vi "diffs.vi"(10 "Array":i32[](array[numeric])) -> (2 "Diffs":i32[](array[numeric]))   [LabVIEW 2014]
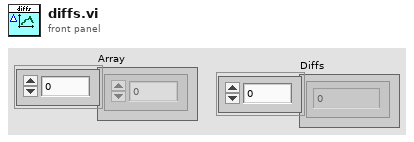
[diagram p1: front panel]
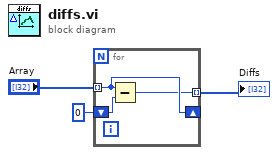
[diagram p0: block diagram]
diagram:
  n1 = for {
    tunnel: "Array" -> [w6] mode=indexing
    shift-right: [w6] -> _
    shift-left: 0 ("Numeric Control") -> [w5]
    tunnel: [w4] -> w1 mode=indexing
    n2 = Subtract(x=w6, y=w5) -> (x-y=w4:i32)
  }
  "Diffs" <- w1
